vi "ReadFile.vi"(0 "template (empty)":path) -> (1 "data":string[][](array[string]), 2 "error out":errorcluster)   [LabVIEW 2020]
uses:
  <vilib>/Utility/NIReport.llb/Report Type.ctl
  <vilib>/addons/_office/excel.llb/Excel Get Data ([str]).vi
  <vilib>/Utility/NIReport.llb/NI_report.lvclass
  <vilib>/Utility/NIReport.llb/Excel/NI_Excel.lvclass
  <vilib>/Utility/NIReport.llb/NI_ReportGenerationCore.lvlib
  <vilib>/addons/_office/NI_ReportGenerationToolkit.lvlib
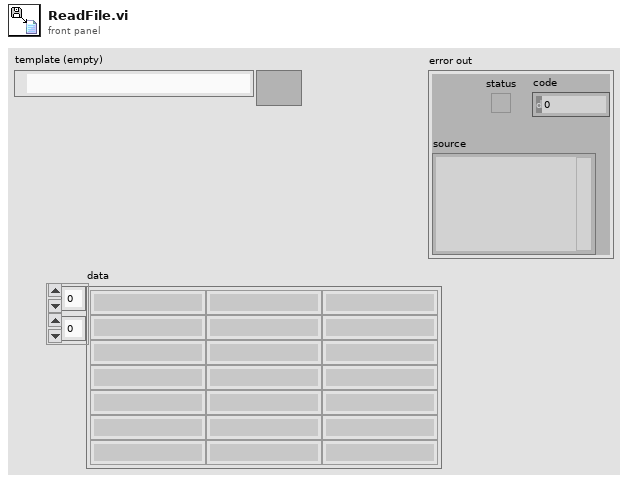
[diagram p1: front panel]
types:
  T1 = typedef "NI_ReportGenerationCore.lvlib/Report Type.ctl" = enum16{"HTML", "Word", "Excel"}
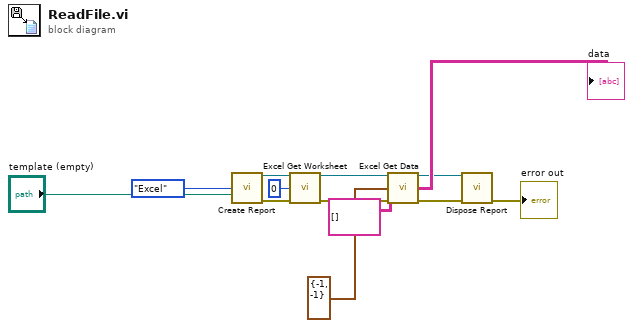
[diagram p0: block diagram]
diagram:
  n1 = call <vilib>:"Create Report.vi"("report type"=Report_Type."Excel", "template (empty)"="template (empty)") -> ("report out"=w11:refnum<class "NI_report.lvclass">, "error out"=w12:errorcluster)  [unwired: 12 in]
  n2 = call <vilib>:"Excel Get Worksheet.vi"("report in"=w11, "worksheet index (0)"=0, "error in (no error)"=w12) -> ("report out"=w8:refnum<class "NI_report.lvclass">, "error out"=w7:errorcluster)  [unwired: 11 in]
  n3 = call-poly <vilib>:"Excel Get Data.vi"("report in"=w8, "data type"=string[][] [], "start (-1, -1)"=cluster{"start row":i32, "start column":i32} {"start row"=-1, "start column"=-1} ("start (0, 0)"), "error in (no error)"=w7) -> ("report out"=w5:refnum<class "NI_report.lvclass">, "data"=→"data":string[][], "error out"=w4:errorcluster)  [unwired: 9 in]
  n4 = call-dynamic "Dispose Report.vi"("report in"=w5, "error in (no error)"=w4) -> ("error out"=→"error out":errorcluster)  [unwired: 13 in]
